vi "test-slew-rate-limiter.vi"(8 "error in (no error)":errorcluster) -> (0 "error out":errorcluster, 3 "All Tests Passed":bool)   [LabVIEW 2019]
uses:
  <vilib>/Rock Robotics/WPI/ThirdParty/JAS_Junk/TrajLib/SlewRateLimiter_New.vi
  <vilib>/Rock Robotics/WPI/ThirdParty/JAS_Junk/TrajLib/SlewRateLimiter_SetRate.vi
  <vilib>/Rock Robotics/WPI/ThirdParty/JAS_Junk/TrajLib/Util_GetTime.vi
  <vilib>/Rock Robotics/WPI/ThirdParty/JAS_Junk/TrajLib/Trajectory_Library.lvlib
panel:
  out "Neg Test Passed":bool
  out "T1 = 0.5":dbl
  out "T0 -- < 2":dbl
  # "Slew Rate Limiter Test"
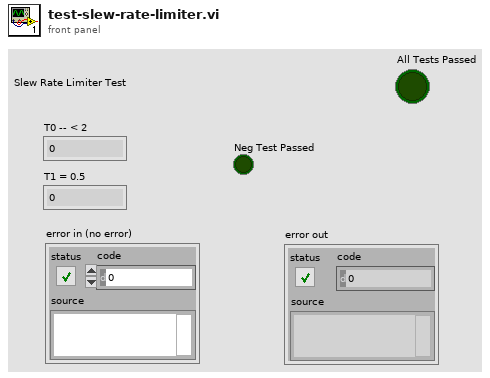
[diagram p1: front panel]
types:
  T1 = typedef "Trajectory_Library.lvlib/SLEW_RATE_LIMITER.ctl" = cluster{"PositiveRateLimit":dbl, "PrevValue":dbl, "PrevTime":dbl, "NegativeRateLimit":dbl}
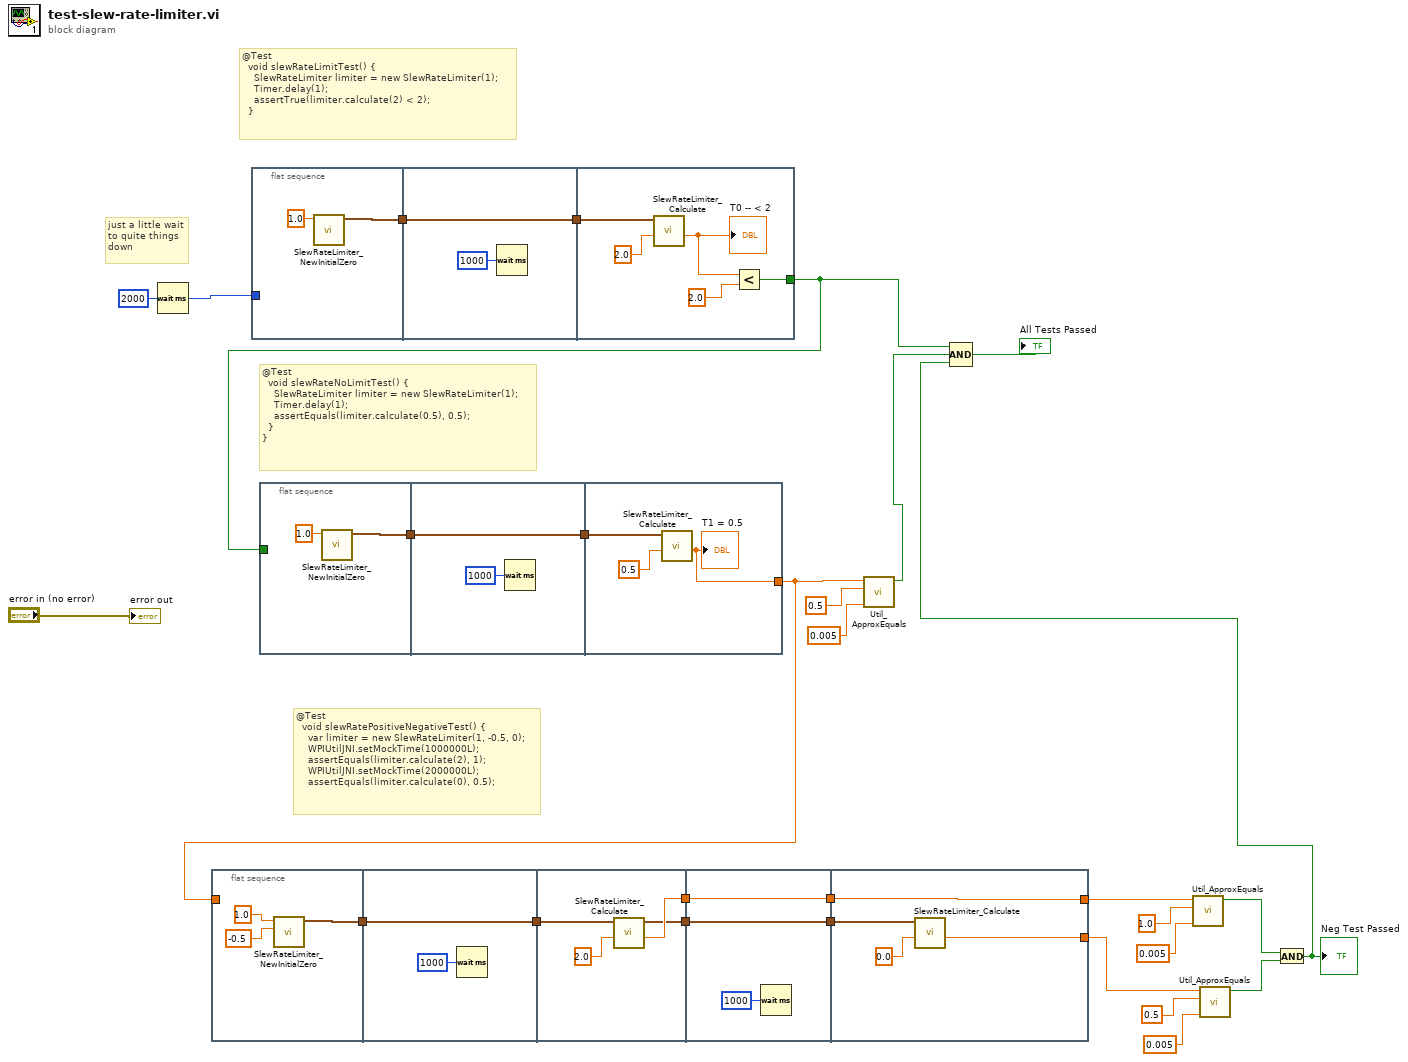
[diagram p0: block diagram]
diagram:
  # "@Test\n  void slewRatePositiveNegativeTest() {\n    var limiter = new SlewRateLimiter(1, -0.5, 0);\n    WPIUtilJNI.setMockTime(1000000L);\n    assertEquals(limiter.calculate(2), 1);\n    WPIUtilJNI.setMockTime(2000000L);\n    assertEquals(limiter.calculate(0), 0.5);"
  # "just a little wait\nto quite things\ndown"
  # "@Test\n  void slewRateNoLimitTest() {\n    SlewRateLimiter limiter = new SlewRateLimiter(1);\n    Timer.delay(1);\n    assertEquals(limiter.calculate(0.5), 0.5);\n  }\n}"
  # "@Test\n  void slewRateLimitTest() {\n    SlewRateLimiter limiter = new SlewRateLimiter(1);\n    Timer.delay(1);\n    assertTrue(limiter.calculate(2) < 2);\n  }"
  n1 = Wait (ms)(milliseconds to wait=u32 2000) -> (millisecond timer value=w19:u32)
  n2 = flat-sequence {
    tunnel: [w30] -> w16
    tunnel: w14 -> [_]
    tunnel: w16 -> [w32]
    tunnel: [w32] -> w15
    tunnel: w15 -> [w36]
    tunnel: [w35] -> w13
    tunnel: [w34] -> w7
    tunnel: w13 -> [w40]
    tunnel: [w40] -> w12
    tunnel: [w38] -> w8
    tunnel: w7 -> [w38]
    tunnel: [w44] -> w9
    tunnel: w12 -> [w44]
    tunnel: w8 -> [w42]
    tunnel: [w41] -> w5
    frame #0 {
      n3 = call <vilib>:"SlewRateLimiter_NewInitialZero.vi"("NegativeRateLimit"=-0.5, "PositiveRateLimit"=1.0 ("RateLimit")) -> ("out SLEW_RATE_LIMITER"=w30:T1)  [unwired: 9 in]
    }
    frame #1 {
      n4 = Wait (ms)(milliseconds to wait=u32 1000) -> ()  [unwired: 1 out]
    }
    frame #2 {
      n5 = call <vilib>:"SlewRateLimiter_Calculate.vi"("Input"=2.0, "in SLEW_RATE_LIMITER"=w36) -> ("Output"=w35:dbl, "out SLEW_RATE_LIMITER"=w34:T1)  [unwired: 8 in]
    }
    frame #3 {
      n6 = Wait (ms)(milliseconds to wait=u32 1000) -> ()  [unwired: 1 out]
    }
    frame #4 {
      n7 = call <vilib>:"SlewRateLimiter_Calculate.vi"("Input"=0.0, "in SLEW_RATE_LIMITER"=w42) -> ("Output"=w41:dbl)  [unwired: 8 in, 1 out]
    }
  }
  n8 = flat-sequence {
    tunnel: [w45] -> w28
    tunnel: w19 -> [_]
    tunnel: w28 -> [w47]
    tunnel: [w47] -> w27
    tunnel: w27 -> [w52]
    tunnel: [w49] -> w17
    frame #0 {
      n9 = call <vilib>:"SlewRateLimiter_NewInitialZero.vi"("PositiveRateLimit"=1.0 ("RateLimit")) -> ("out SLEW_RATE_LIMITER"=w45:T1)  [unwired: 10 in]
    }
    frame #1 {
      n10 = Wait (ms)(milliseconds to wait=u32 1000) -> ()  [unwired: 1 out]
    }
    frame #2 {
      n11 = call <vilib>:"SlewRateLimiter_Calculate.vi"("Input"=2.0, "in SLEW_RATE_LIMITER"=w52) -> ("Output"=w51:dbl)  [unwired: 8 in, 1 out]
      "T0 -- < 2" <- w51
      n12 = Less?(x=w51, y=2.0) -> (x < y?=w49:bool)
    }
  }
  n13 = flat-sequence {
    tunnel: [w54] -> w26
    tunnel: w17 -> [_]
    tunnel: w26 -> [w56]
    tunnel: [w56] -> w25
    tunnel: w25 -> [w59]
    tunnel: [w58] -> w14
    frame #0 {
      n14 = call <vilib>:"SlewRateLimiter_NewInitialZero.vi"("PositiveRateLimit"=1.0 ("RateLimit")) -> ("out SLEW_RATE_LIMITER"=w54:T1)  [unwired: 10 in]
    }
    frame #1 {
      n15 = Wait (ms)(milliseconds to wait=u32 1000) -> ()  [unwired: 1 out]
    }
    frame #2 {
      n16 = call <vilib>:"SlewRateLimiter_Calculate.vi"("Input"=0.5, "in SLEW_RATE_LIMITER"=w59) -> ("Output"=w58:dbl)  [unwired: 8 in, 1 out]
      "T1 = 0.5" <- w58
    }
  }
  n17 = call <vilib>:"Util_ApproxEquals.vi"("Tolerance"=0.005, "Value 2"=0.5, "Value 1"=w14) -> ("ApproxEquals"=w23:bool)  [unwired: 8 in]
  n18 = call <vilib>:"Util_ApproxEquals.vi"("Tolerance"=0.005, "Value 2"=1.0, "Value 1"=w9) -> ("ApproxEquals"=w3:bool)  [unwired: 8 in]
  n19 = call <vilib>:"Util_ApproxEquals.vi"("Tolerance"=0.005, "Value 2"=0.5, "Value 1"=w5) -> ("ApproxEquals"=w2:bool)  [unwired: 8 in]
  n20 = And(x=w3, y=w2) -> (x .and. y?=w1:bool)
  "Neg Test Passed" <- w1
  n21 = Compound Arithmetic op=AND(w17, w23, w1) -> (→"All Tests Passed":bool)
  "error out" <- "error in (no error)"
